vi "_test_parse_build.vi"() -> ()   [LabVIEW 2013, in "CfgManager.Text.lvlib" / "ConfigManager.Text.INI.lvclass"]
uses:
  ConfigManager.Text.INI.lvclass
panel:
  out "PASS":bool
  out "Input String":string
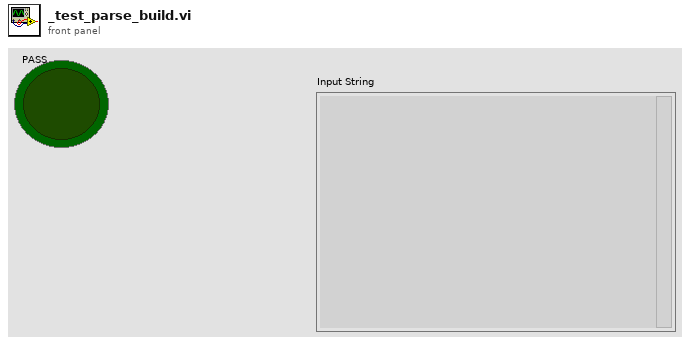
[diagram p1: front panel]
types:
  T1 = typedef "CfgManager.Text.lvlib/ConfigManager.Text.lvclass/Dictionary Payload -- cluster.ctl" = cluster{"Value":string, "Comment":string, "stack position":i32}
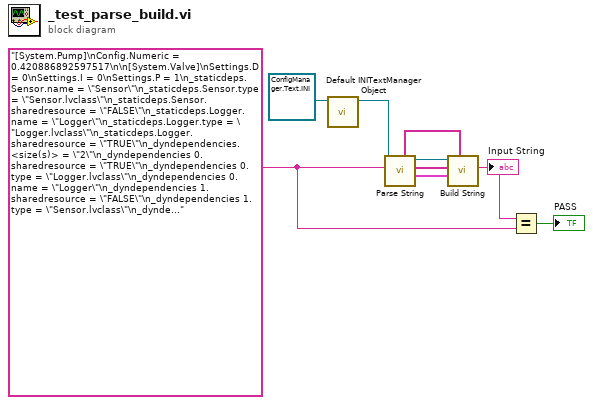
[diagram p0: block diagram]
diagram:
  w4 = "[System.Pump]\nConfig.Numeric = 0.420886892597517\n\n[System.Valve]\nSettings.D = 0\nSettings.I = 0\nSettings.P = 1\n_staticdeps.Sensor.name = \"Sensor\"\n_staticdeps.Sensor.type = \"Sensor.lvclass\"\n_staticdeps.Sensor.sharedresource = \"FALSE\"\n_staticdeps.Logger.name = \"Logger\"\n_staticdeps.Logger.type = \"Logger.lvclass\"\n_staticdeps.Logger.sharedresource = \"TRUE\"\n_dyndependencies.<size(s)> = \"2\"\n_dyndependencies 0.sharedresource = \"TRUE\"\n_dyndependencies 0.type = \"Logger.lvclass\"\n_dyndependencies 0.name = \"Logger\"\n_dyndependencies 1.sharedresource = \"FALSE\"\n_dyndependencies 1.type = \"Sensor.lvclass\"\n_dyndependencies 1.name = \"Sensor\"\n\n[System.Sensor]\nnumerics = \"<size(s)=2> 3.14159 2.7818\"" ("Input String")
  n1 = call-dynamic "Default INITextManager Object.vi"("CfgManager.Text.INI in"=refnum<class "ConfigManager.Text.INI.lvclass"> refnum ("CfgManager.Text.lvlib:ConfigManager.Text.INI.lvclass")) -> ("CfgManager.Text.INI out"=w2:refnum<class "ConfigManager.Text.INI.lvclass">)  [unwired: 10 in]
  n2 = call-dynamic "Parse String.vi"("Input String"=w4, "ConfigManager.Text.INI in"=w2) -> ("Content"=w6:T1[], "Keys"=w7:string[], "ConfigManager.Text.INI out"=w9:refnum<class "ConfigManager.Text.INI.lvclass">, "Section"=w8:string[])  [unwired: 5 in, 1 out]
  n3 = call-dynamic "Build String.vi"("Section"=w8, "Content"=w6, "Keys"=w7, "ConfigManager.Text in"=w9) -> ("Input String"=w5:string)  [unwired: 5 in, 2 out]
  "Input String" <- w5
  n4 = Equal?(x=w5, y=w4) -> (x = y?=→"PASS":bool)
